vi "Handle Routing Channel State Change.vi"(4 "force update":bool, 5 "Routing and Faulting Custom Device Ref":T1 format="%.0x", 6 "init index":bool=TRUE, 7 "Channel Editor State":T2={"Modules and Connections"=[{" Module Path"="", "Short Module Path"="", "Product Name"="", "Possible Connections"=[], "Missing"=FALSE}, {" Module Path"="", "Short Module Path"="", "Product Name"="", "Possible Connections"=[], "Missing"=FALSE}], "Alias Mappings UI"=[], "Mappings by Module UI"=[]}, 8 "error in (no error)":errorcluster, 9 "State":string, 10 "Routing Channel Page Controls":T8, 11 "Routing Channel Ref in":T1 format="%.0x") -> (0 "error out":errorcluster, 3 "Routing Channel Ref out":T1 format="%.0x")   [LabVIEW 2020, in "Routing and Faulting System Explorer.lvlib"]
uses:
  Routing and Faulting System Explorer.lvlib
  <vilib>/NI VeriStand/Custom Device API/Custom Device Item Ref.ctl
  Routing Channel Page Controls.ctl
  Channel Editor State.ctl
  Possible Connections.ctl
  Shared/Routing and Faulting Hardware API/Types/Possible Connections for Endpoint.ctl
  Shared/Alias Mapping.ctl
  Shared/Alias Endpoint.ctl
  Alias Map by Module.ctl
  Shared/Constants.vi
  Scripting/Routing and Faulting Scripting.lvlib
  Shared/Routing and Faulting Shared.lvlib
  <vilib>/NI VeriStand/Custom Device API/Custom Device API.lvlib
  Shared/Routing and Faulting Hardware API/Routing and Faulting Hardware API.lvlib
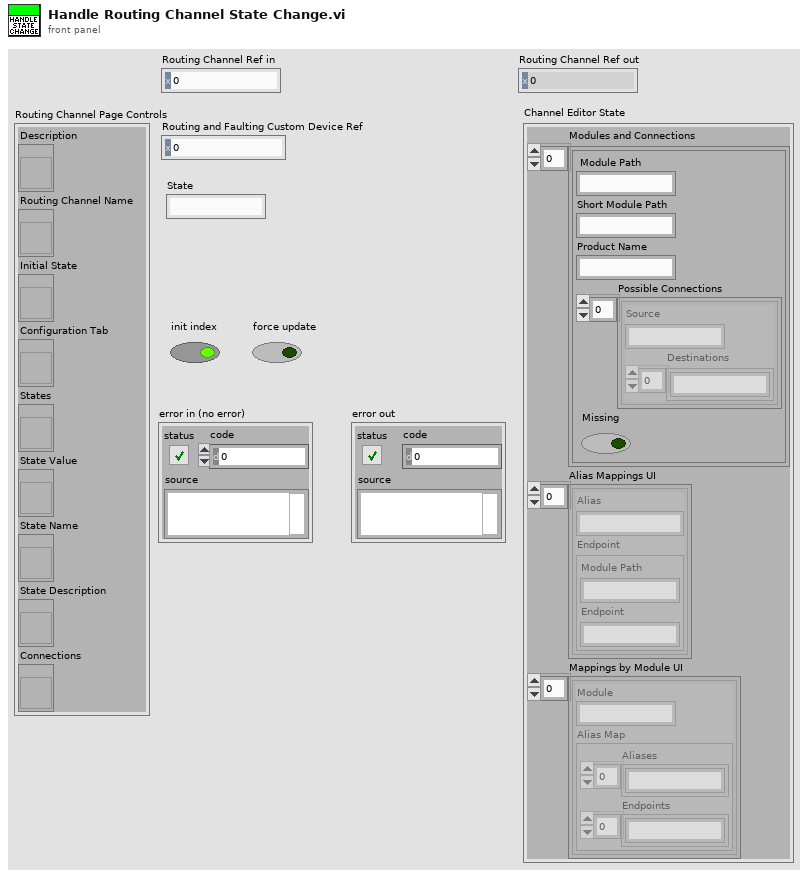
[diagram p1: front panel]
types:
  T1 = typedef "Custom Device API.lvlib/Custom Device Item Ref.ctl" = u64
  T2 = typedef "Routing and Faulting System Explorer.lvlib/Channel Editor State.ctl" = cluster{"Modules and Connections":T3[], "Alias Mappings UI":T5[], "Mappings by Module UI":T7[]}
  T3 = typedef "Routing and Faulting System Explorer.lvlib/Possible Connections.ctl" = cluster{" Module Path":string, "Short Module Path":string, "Product Name":string, "Possible Connections":T4[], "Missing":bool}
  T4 = typedef "Routing and Faulting Hardware API.lvlib/Possible Connections for Endpoint.ctl" = cluster{"Source":string, "Destinations":string[]}
  T5 = typedef "Routing and Faulting Shared.lvlib/Alias Mapping.ctl" = cluster{"Alias":string, "Endpoint":T6}
  T6 = typedef "Routing and Faulting Shared.lvlib/Alias Endpoint.ctl" = cluster{"Module Path":string, "Endpoint":string}
  T7 = typedef "Routing and Faulting System Explorer.lvlib/Alias Map by Module.ctl" = cluster{"Module":string, "Alias Map":cluster{"Aliases":string[], "Endpoints":string[]}}
  T8 = typedef "Routing and Faulting System Explorer.lvlib/Routing Channel Page Controls.ctl" = cluster{"Description":refnum<vi>, "Routing Channel Name":refnum<vi>, "Initial State":refnum<vi>, "Configuration Tab":refnum<vi>, "States":refnum<vi>, "State Value":refnum<vi>, "State Name":refnum<vi>, "State Description":refnum<vi>, "Connections":refnum<vi>}
  T9 = typedef "Routing and Faulting Shared.lvlib/Routing State.ctl" = cluster{"Name":string, "Description":string, "Value":i32, "Connection List":T10[]}
  T10 = typedef "Routing and Faulting Shared.lvlib/Connection.ctl" = cluster{"Module":string, "Source":string, "Destination":string}
  T11 = typedef "Routing and Faulting System Explorer.lvlib/State-Value Row.ctl" = cluster{"State":string, "State Value":string}
  T12 = typedef "Routing and Faulting System Explorer.lvlib/Connection Row.ctl" = cluster{"Source":string, "Destination":string, "Edit":bool, "Remove":bool}
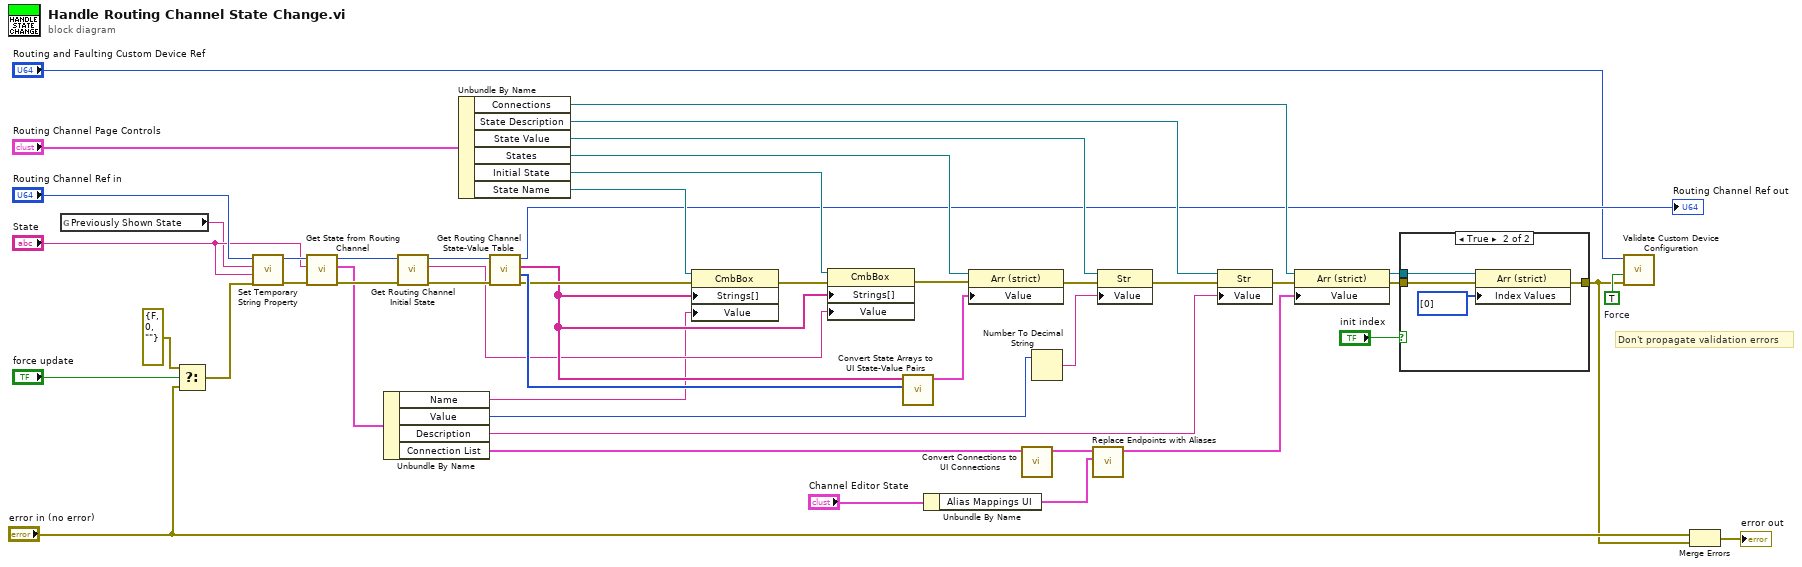
[diagram p0: block diagram]
diagram:
  w2 = TRUE  # Force
  # "Don't propagate validation errors"
  n1 = global read "Constants.vi" "Previously Shown State"() -> (w5:string)
  n2 = Select(t=errorcluster {"status"=FALSE, "code"=0, "source"=""}, s="force update", f="error in (no error)") -> (s? t:f=w9:errorcluster)
  n3 = call "Set Temporary String Property.vi"("error in (no error)"=w9, "value"="State", "property name"=w5, "Item Ref in"="Routing Channel Ref in") -> ("error out"=w10:errorcluster, "Item Ref out"=w7:T1)  [unwired: 6 in]
  n4 = call "Get State from Routing Channel.vi"("error in"=w10, "state"="State", "routing channel in"=w7) -> ("error out"=w39:errorcluster, "state and connections"=w36:T9, "routing channel out"=w21:T1)  [unwired: 6 in]
  n5 = Unbundle By Name(w36) -> ("Name"=w13:string, "Value"=w48:i32, "Description"=w43:string, "Connection List"=w46:T10[])
  n6 = call "Get Routing Channel Initial State.vi"("error in"=w39, "routing channel in"=w21) -> ("error out"=w22:errorcluster, "initial state"=w18:string, "routing channel out"=w20:T1)  [unwired: 7 in]
  n7 = Unbundle By Name("Routing Channel Page Controls") -> ("Connections"=w30:refnum<vi>, "State Description"=w42:refnum<vi>, "State Value"=w14:refnum<vi>, "States"=w33:refnum<vi>, "Initial State"=w17:refnum<vi>, "State Name"=w32:refnum<vi>)
  n8 = call "Get Routing Channel State-Value Table.vi"("error in"=w22, "routing channel in"=w20) -> ("error out"=w35:errorcluster, "state values"=w38:i32[], "state names"=w19:string[], "routing channel out"=→"Routing Channel Ref out":T1)  [unwired: 6 in]
  n9 = property class="CmbBox"(reference=w32, error in=w35, "Strings[]"=w19, "Value"=w13) -> (error out=w16:errorcluster)  [unwired: 1 out]
  n10 = property class="CmbBox"(reference=w17, error in=w16, "Strings[]"=w19, "Value"=w18) -> (error out=w15:errorcluster)  [unwired: 1 out]
  n11 = call "Convert State Arrays to UI State-Value Pairs.vi"("State Values"=w38, "State Names"=w19) -> ("State-Value Pairs"=w37:T11[])  [unwired: 9 in]
  n12 = Unbundle By Name("Channel Editor State") -> ("Alias Mappings UI"=w11:T5[])
  n13 = property class="Arr (strict)"(reference=w33, error in=w15, "Value"=w37) -> (error out=w34:errorcluster)  [unwired: 1 out]
  n14 = call "Convert Connections to UI Connections.vi"("Connection List"=w46) -> ("UI Connections List"=w41:T12[])  [unwired: 10 in]
  n15 = Number To Decimal String(number=w48) -> (decimal integer string=w31:string)  [unwired: 1 in]
  n16 = call "Replace Endpoints with Aliases.vi"("Alias Mappings"=w11, "UI Connections List in"=w41) -> ("UI Connections List out"=w40:T12[])  [unwired: 9 in]
  n17 = property class="Str"(reference=w14, error in=w34, "Value"=w31) -> (error out=w45:errorcluster)  [unwired: 1 out]
  n18 = property class="Str"(reference=w42, error in=w45, "Value"=w43) -> (error out=w44:errorcluster)  [unwired: 1 out]
  n19 = property class="Arr (strict)"(reference=w30, error in=w44, "Value"=w40) -> (reference out=w29:refnum<vi>, error out=w28:errorcluster)
  n20 = case shown="True" "init index" {
    tunnel: w29 -> [_ w52]
    tunnel: w28 -> [w49 w51]
    tunnel: [w49 w50] -> w1
    frame False {
    }
    frame True {
      n21 = property class="Arr (strict)"(reference=w52, error in=w51, "Index Values"=u32[] [0]) -> (error out=w50:errorcluster)  [unwired: 1 out]
    }
  }
  n22 = call "Validate Custom Device Configuration.vi"("error in (no error)"=w1, "Force Validation (F)"=w2, "Routing and Faulting Custom Device Ref"="Routing and Faulting Custom Device Ref") -> ()  [unwired: 6 in, 3 out]
  n23 = Merge Errors("error in (no error)", w1) -> (→"error out":errorcluster)
